vi "Find Msgs.vi"(11 "Base Actor in":refnum<class "Base Actor.lvclass">) -> (2 "Msgs":T1)   [LabVIEW 2020, in "jettl.lvlib" / "BaseActor.lvlib" / "Base Actor.lvclass"]
uses:
  Base Actor.lvclass
  Base Actor.lvclass/Base Actor.ctl
  C:/jettl-harness/repos/jettl/src/jettl/jettl/MediatorActor/Base Actor/Base Actor.lvclass
  C:/jettl-harness/repos/jettl/src/jettl/jettl/Actor/Actor.lvclass
  jettl.lvlib
  Message/Message.lvclass
  MessageSet.ctl
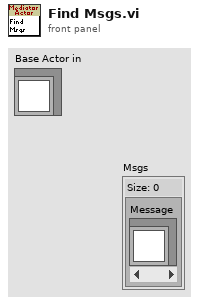
[diagram p1: front panel]
types:
  T1 = typedef "jettl.lvlib/MessageSet.ctl" = set{refnum<class "Message.lvclass">}
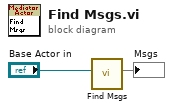
[diagram p0: block diagram]
diagram:
  n1 = call "Find Msgs.vi"("X Actor.lvclass"="Base Actor in") -> ("Msgs"=→"Msgs":T1)  [unwired: 10 in]
